vi "Lecture fichier texte.vi"(3 "séparateur (Tab)":string, 4 "file path (dialog if empty)":path caption="chemin du fichier (boîte de dialogue si vide)") -> (0 "Table":string[][](table), 1 "file path (dialog if empty) 2":path caption="chemin du fichier (boîte de dialogue si vide)")   [LabVIEW 2013]
panel:
  in  "Type tableau de chaine":string[][](array[string])
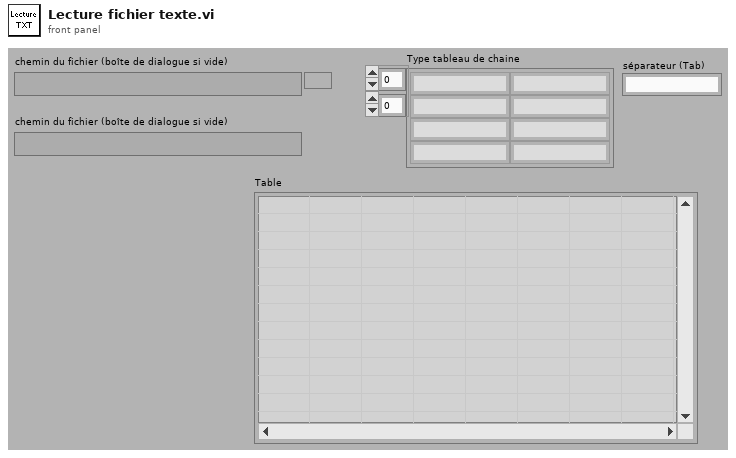
[diagram p1: front panel]
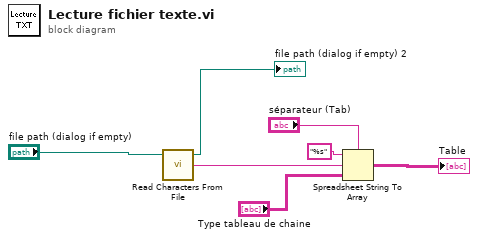
[diagram p0: block diagram]
diagram:
  n1 = call <vilib>:"Read Characters From File.vi"("file path (dialog if empty)"="file path (dialog if empty)") -> ("new file path (NotAPath if cancelled)"=→"file path (dialog if empty) 2":path, "character string"=w6:string)  [unwired: 5 in, 2 out]
  n2 = Spreadsheet String To Array(delimiter (Tab)="séparateur (Tab)", format string="%s" ("chaîne de format"), spreadsheet string=w6, array type (2D Dbl)="Type tableau de chaine") -> (array=→"Table":string[][])
